vi "Warning.vi"(8 "error in (no error)":errorcluster, 11 "Error info":T1) -> (0 "error out":errorcluster)   [LabVIEW 2017, in "Error.lvlib"]
doc: "Write data to main coms q for module (generic)"
uses:
  Error.lvlib
  ctl/ErrorInfo.ctl
  ctl/MainData.ctl
  ctl/MainStates.ctl
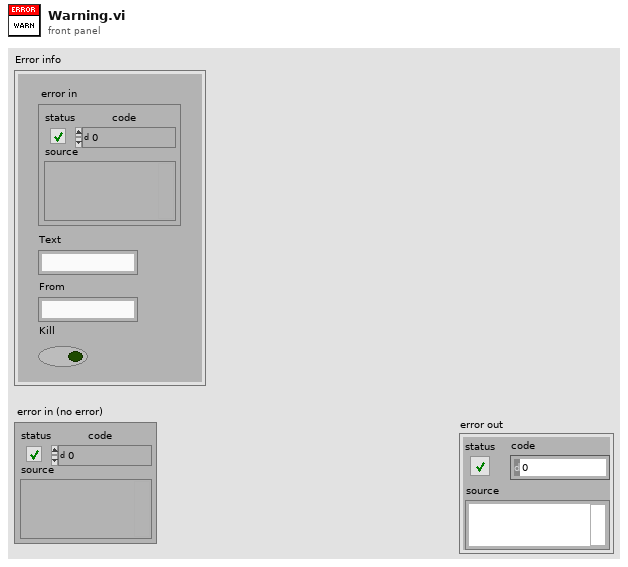
[diagram p1: front panel]
types:
  T1 = typedef "Error.lvlib/ErrorInfo.ctl" = cluster{"error in":errorcluster, "Text":string, "From":string, "Kill":bool}
  T2 = typedef "Error.lvlib/MainStates.ctl" = enum16{"Timeout", "Error", "Exit", "Init", "ClassError", "LogError", "Shutdown", "Warning"}
  T3 = typedef "Error.lvlib/MainData.ctl" = cluster{"State":T2, "Variant":variant}
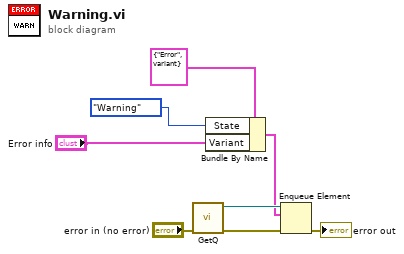
[diagram p0: block diagram]
diagram:
  n1 = call "GetQ.vi"("error in (no error)"="error in (no error)") -> ("error out"=w7:errorcluster, "Q out"=w8:refnum<queue>)  [unwired: 9 in]
  n2 = Bundle By Name(cluster=T3 {"State"=enum."Error", "Variant"=variant} ("Data"), "State"=MainStates."Warning", "Variant"="Error info") -> (w4:T3)
  n3 = Enqueue Element(queue=w8, element=w4, error in (no error)=w7) -> (error out=→"error out":errorcluster)  [unwired: 1 in, 2 out]
